vi "findItem.vi"(6 "storageSheets":T1, 8 "error in (no error)":errorcluster, 9 "item":string, 10 "itemColumn":T2, 11 "reference in":refnum<class "Items Controller.lvclass">) -> (0 "error out":errorcluster, 1 "found!":bool, 2 "indexElements":i32[](array[numeric]), 3 "reference out":refnum<class "Items Controller.lvclass">)   [LabVIEW 2015, in "Items Controller.lvclass"]
uses:
  Items Controller.lvclass
  itemsColumn.ctl
  storageSheets.ctl
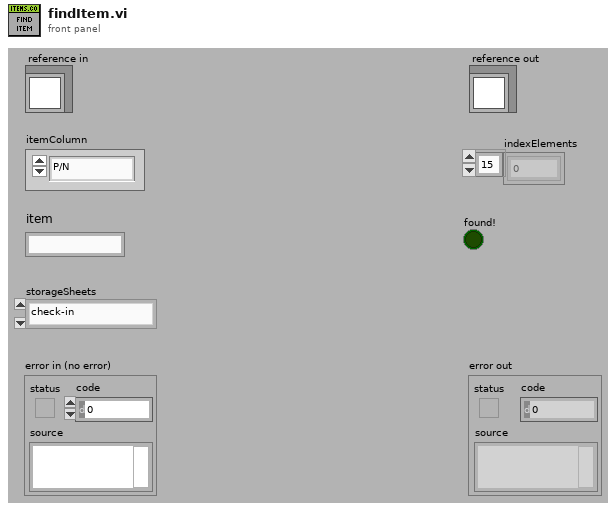
[diagram p1: front panel]
types:
  T1 = typedef "Items Controller.lvclass/storageSheets.ctl" = enum16{"check-in", "check-out", "storage"}
  T2 = typedef "Items Controller.lvclass/itemsColumn.ctl" = enum16{"P/N", "S/N", "Description"}
  T3 = typedef "Items Controller.lvclass/ObjectAttributesRef.ctl" = refnum<data-value>
  T4 = typedef "Items Controller.lvclass/ObjectAttributes.ctl" = cluster{"MyAttribute":dbl, "data":string[][][], "file_controller_ref":refnum<class "File Controller.lvclass">, "checkIN_ref":refnum<class "checkIN.lvclass">, "checkOUT_ref":refnum<class "checkOUT.lvclass">, "item_ref":refnum<class "item.lvclass">}
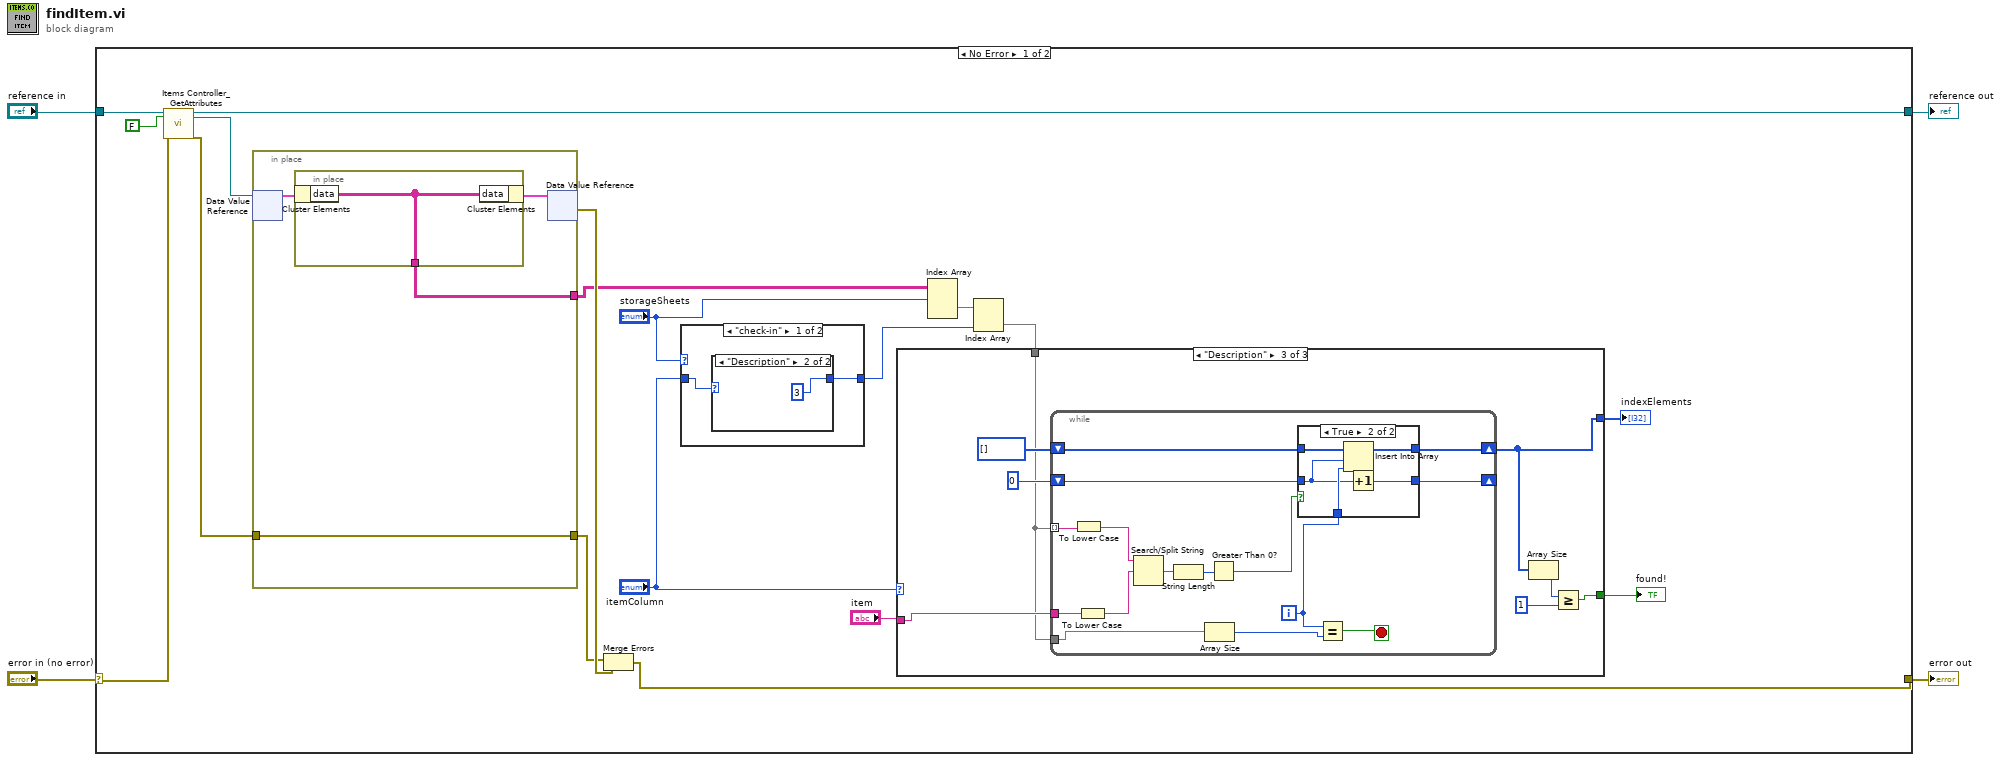
[diagram p0: block diagram]
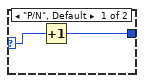
[diagram p2: hidden frame]
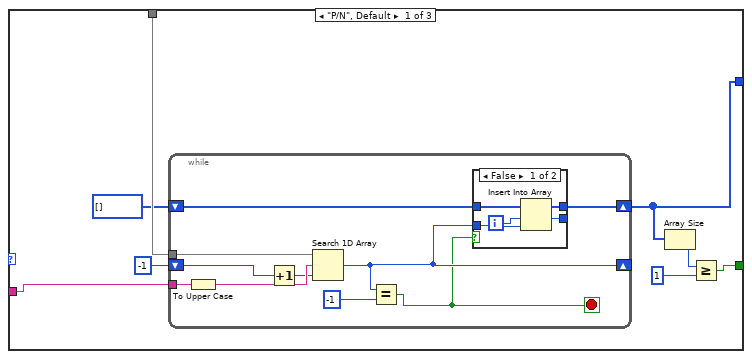
[diagram p4: hidden frame]
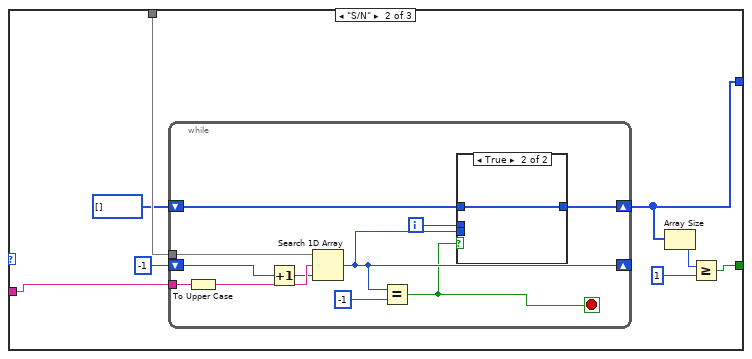
[diagram p6: hidden frame]
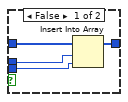
[diagram p7: hidden frame]
diagram:
  n1 = case shown="No Error" "error in (no error)" {
    selector: "error in (no error)" -> [w17 w113]
    tunnel: [w22 w113] -> w3
    tunnel: [w15 w112] -> w1
    tunnel: "reference in" -> [w19 w112]
    frame No Error {
      n2 = call "Items Controller_GetAttributes.vi"("reference in"=w19, "return data? (T)"=FALSE, "error in (no error)"=w17) -> ("reference out"=w15:refnum<class "Items Controller.lvclass">, "attributes ref"=w14:T3, "error out"=w16:errorcluster)  [unwired: 13 in, 1 out]
      n3 = in-place {
        in-place-border: w16 -> [w108]
        in-place-border: [w108] -> w20
        in-place-border: [w107] -> w12
        n4 = in-place-dvr #1(w14) -> (w109:T4)  [unwired: 1 out]
        n5 = in-place {
          in-place-border: [w111] -> w107
          n6 = in-place-cluster #2(w109) -> ("data"=w111:string[][][])
          n7 = in-place-cluster #2("data"=w111) -> (w110:T4)
        }
        n8 = in-place-dvr #1(w110) -> (w21:errorcluster)  [unwired: 1 out]
      }
      n9 = Merge Errors(w20, w21) -> (w22:errorcluster)
      n10 = case shown="\"check-in\"" "storageSheets" {
        tunnel: "itemColumn" -> [w24 w28]
        tunnel: [w23 w28] -> w6
        frame "check-in" {
          n11 = case shown="\"Description\"" w24 {
            selector: w24 -> [w26 _]
            tunnel: [w25 3] -> w23
            frame "P/N", Default {
              n12 = Increment(x=w26) -> (x+1=w25:T2)
            }
            frame "Description" {
            }
          }
        }
        frame "check-out", Default {
        }
      }
      n13 = Index Array(array=w12, index (dim 0)="storageSheets") -> (element=w13:string[][])  [unwired: 2 in]
      n14 = Index Array(array=w13, index (col)=w6) -> (element=w11:string[])  [unwired: 1 in]
      n15 = case shown="\"Description\"" "itemColumn" {
        tunnel: "item" -> [w35 w59 w84]
        tunnel: w11 -> [w36 w60 w77]
        tunnel: [w31 w55 w81] -> w10
        tunnel: [w32 w56 w82] -> w5
        frame "P/N", Default {
          n16 = while {
            tunnel: w36 -> [w44]
            tunnel: w35 -> [w46]
            shift-right: [w40] -> _
            shift-left: -1 ("index of element") -> [w43]
            shift-right: [w39] -> w32
            shift-left: i32[] [] -> [w42]
            i -> [w41]
            stop <- w37 stop-if-true
            n17 = To Upper Case(1:w46) -> (0:w45:string)
            n18 = Increment(x=w43) -> (x+1=w38:i32)
            n19 = Search 1D Array(1D array=w44, element=w45, start index (0)=w38) -> (index of element=w40:i32)
            n20 = Equal?(x=w40, y=-1) -> (x = y?=w37:bool)
            n21 = case shown="False" w37 {
              tunnel: w42 -> [w51 w52]
              tunnel: w41 -> [w50 _]
              tunnel: w40 -> [w49 _]
              tunnel: [w48 w52] -> w39
              frame False {
                n22 = Insert Into Array(array=w51, index=w50, new element=w49) -> (w48:i32[])
              }
              frame True {
              }
            }
          }
          n23 = Array Size(array=w32) -> (size(s)=w30:i32)
          n24 = Greater Or Equal?(x=w30, y=1) -> (x >= y?=w31:bool)
        }
        frame "S/N" {
          n25 = while {
            tunnel: w60 -> [w68]
            tunnel: w59 -> [w70]
            shift-right: [w64] -> _
            shift-left: -1 ("index of element") -> [w67]
            shift-right: [w63] -> w56
            shift-left: i32[] [] -> [w66]
            i -> [w65]
            stop <- w61 stop-if-true
            n26 = To Upper Case(1:w70) -> (0:w69:string)
            n27 = Increment(x=w67) -> (x+1=w62:i32)
            n28 = Search 1D Array(1D array=w68, element=w69, start index (0)=w62) -> (index of element=w64:i32)
            n29 = Equal?(x=w64, y=-1) -> (x = y?=w61:bool)
            n30 = case shown="True" w61 {
              tunnel: w66 -> [w75 w76]
              tunnel: w65 -> [w74 _]
              tunnel: w64 -> [w73 _]
              tunnel: [w72 w76] -> w63
              frame False {
                n31 = Insert Into Array(array=w75, index=w74, new element=w73) -> (w72:i32[])
              }
              frame True {
              }
            }
          }
          n32 = Array Size(array=w56) -> (size(s)=w54:i32)
          n33 = Greater Or Equal?(x=w54, y=1) -> (x >= y?=w55:bool)
        }
        frame "Description" {
          n34 = while {
            tunnel: w77 -> [w96] mode=indexing
            tunnel: w84 -> [w97]
            shift-right: [w98] -> w82
            shift-left: i32[] [] -> [w99]
            shift-right: [w89] -> _
            shift-left: 0 ("index of element") -> [w90]
            tunnel: w77 -> [w88]
            i -> [w85]
            stop <- w86 stop-if-true
            n35 = To Lower Case(string=w96) -> (all lower case string=w92:string)
            n36 = To Lower Case(string=w97) -> (all lower case string=w93:string)
            n37 = Search/Split String(string=w92, search string/char (-)=w93) -> (match + rest of string=w95:string)  [unwired: 1 in, 2 out]
            n38 = String Length(string=w95) -> (length=w94:i32)
            n39 = Array Size(array=w88) -> (size(s)=w87:i32)
            n40 = Greater Than 0?(x=w94) -> (x > 0?=w91:bool)
            n41 = case shown="True" w91 {
              tunnel: w99 -> [w100 w106]
              tunnel: [w100 w105] -> w98
              tunnel: w90 -> [w101 w103]
              tunnel: w85 -> [_ w104]
              tunnel: [w101 w102] -> w89
              frame False {
              }
              frame True {
                n42 = Insert Into Array(array=w106, index=w103, new element=w104) -> (w105:i32[])
                n43 = Increment(x=w103) -> (x+1=w102:i32)
              }
            }
            n44 = Equal?(x=w85, y=w87) -> (x = y?=w86:bool)
          }
          n45 = Array Size(array=w82) -> (size(s)=w80:i32)
          n46 = Greater Or Equal?(x=w80, y=1) -> (x >= y?=w81:bool)
        }
      }
      "found!" <- w10
      "indexElements" <- w5
    }
    frame Error {
    }
  }
  "error out" <- w3
  "reference out" <- w1
